vi "Main.vi"(8 "error in (no error)":errorcluster, 11 "ModuleAdmin":refnum<class "ModuleAdmin.lvclass">) -> ()   [LabVIEW 2014, in "OutputToFileModule.lvlib"]
uses:
  OutputToFileModule.lvlib
  <userlib>/NIST/ModuleAdminLib/ModuleAdmin/ModuleAdmin.lvclass
  PublicAPI/Arguments/Requests/clStopArgument.ctl
  <userlib>/NIST/ModuleAdminLib/ModuleAdmin/ModuleAdmin.lvclass/ModuleAdmin.ctl
  OutputToFilePlugins/OutputToFileBasePlugin/OutputToFileBasePlugin.lvclass
  <userlib>/NIST/BaseClasses/BasePlugin_class/BasePlugin.lvclass/BasePlugin.ctl
  OutputToFilePlugins/OutputToFileBasePlugin/OutputToFileBasePlugin.lvclass/OutputToFileBasePlugin.ctl
  EventPlugins/EventPluginBaseClass/TypeDefs/clEvtReportArray.ctl
  EventPlugins/EventPluginBaseClass/TypeDefs/clEvtReport.ctl
  NetworkImpairmentModule/PublicAPI/Arguments/Broadcasts/dblPktLoss.ctl
  NetworkImpairmentModule/PublicAPI/Arguments/Broadcasts/dblNetworkTime.ctl
  OutputToFilePlugins/OutputToFileBasePlugin/Typedefs/PmuCfgOpt.ctl
  <vilib>/Utility/error.llb/DialogType.ctl
  <userlib>/NIST/ModuleAdminLib/ModuleAdmin/Accessors/Read ShowPanel_.vi
  <userlib>/NIST/ModuleAdminLib/ModuleAdmin/Accessors/Write ShowPanel_.vi
  <userlib>/NIST/BaseClasses/BasePlugin_class/Accessors/Write PluginIniFilePath.vi
  <userlib>/NIST/BaseClasses/BasePlugin_class/Accessors/Read PluginIniFilePath.vi
  OutputToFilePlugins/OutputToFileBasePlugin/Accessors/Read clConfigOptions.vi
  OutputToFilePlugins/OutputToFileBasePlugin/Accessors/Read OutputPath.vi
  OutputToFilePlugins/OutputToFileBasePlugin/Accessors/Write clEvtReportArray.vi
  OutputToFilePlugins/OutputToFileBasePlugin/Accessors/Write PmuImpairRptArray.vi
  OutputToFilePlugins/OutputToFileBasePlugin/Accessors/Write OutputPath.vi
  OutputToFilePlugins/OutputToFileBasePlugin/Accessors/Write dblPktLoss.vi
  OutputToFilePlugins/OutputToFileBasePlugin/Accessors/Write dblNetworkTime.vi
  OutputToFilePlugins/OutputToFileBasePlugin/Accessors/Write clConfigOptions.vi
  OutputToFilePlugins/OutputToFileBasePlugin/Accessors/Read EvtRptArray.vi
  OutputToFilePlugins/OutputToFileBasePlugin/Accessors/Read PmuImpairRptArray.vi
  <userlib>/NIST/ModuleAdminLib/ModuleAdmin/Accessors/Read CloneRegRef.vi
  <vilib>/Utility/error.llb/Error Cluster From Error Code.vi
  <vilib>/Utility/file.llb/Write To Spreadsheet File (string).vi
  <vilib>/ErrorRing/Error Ring.xnode
  <userlib>/NIST/ModuleAdminLib/CloneRegistration/CloneRegistration.lvclass
  <userlib>/NIST/ModuleAdminLib/ModuleAdmin.lvlib
  <userlib>/NIST/BaseClasses/Object_class/BaseObject.lvclass
  EventPlugins/EventPluginBaseClass/EventPluginBaseClass.lvclass
  NetworkImpairmentModule/NetworkImpairmentModule.lvlib
panel:
  out "error out":errorcluster
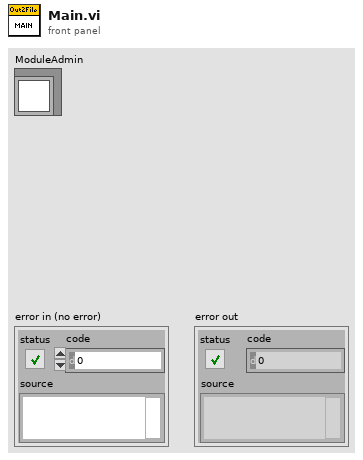
[diagram p1: front panel]
types:
  T1 = typedef "OutputToFileModule.lvlib/clRequestEvents.ctl" = cluster{"StopRequest":refnum<user-event>, "LoadPluginRequest":refnum<user-event>, "ReadPathToPluginRequest":refnum<user-event>, "WriteEvtRptRequest":refnum<user-event>, "WritePmuImpairRptRequest":refnum<user-event>, "WriteNetTimeRequest":refnum<user-event>, "WritePktLossRequest":refnum<user-event>, "WritePmuConfigRequest":refnum<user-event>, "ReadPmuConfigRequest":refnum<user-event>, "WriteOutPathRequest":refnum<user-event>, "ReadOutPathRequest":refnum<user-event>, "WriteFlagImpairRequest":refnum<user-event>, "OutputRefFileRequest":refnum<user-event>, "OutputImpairedFileRequest":refnum<user-event>, "OutputErrorDataRequest":refnum<user-event>, "OpenConfigRequest":refnum<user-event>, "ShowPanel":refnum<user-event>}
  T2 = typedef "OutputToFileModule.lvlib/clBroadcastEvents.ctl" = cluster{"DidInit":refnum<user-event>, "StatusUpdate":refnum<user-event>, "ErrorReport":refnum<user-event>, "DidStop":refnum<user-event>, "PathToPlugin":refnum<user-event>, "PmuConfig":refnum<user-event>, "OutputPath":refnum<user-event>}
  T3 = typedef "OutputToFileModule.lvlib/clStopArgument.ctl" = cluster{"Exit via Stop Module Req?":bool, "Wait for Module to stop?":bool, "ModuleAdmin":refnum<class "ModuleAdmin.lvclass">}
  T4 = enum32{"Invalid", "Standard", "Closed", "Hidden", "Minimized", "Maximized"}
  T5 = typedef "EventPlugins.lvlib/EventPluginBaseClass.lvclass/clEvtReportArray.ctl" = T6[]
  T6 = typedef "EventPlugins.lvlib/EventPluginBaseClass.lvclass/clEvtReport.ctl" = cluster{"Timestamp":dbl, "Synx":cdb[], "Freq":dbl, "ROCOF":dbl, "ID":i16}
  T7 = typedef "OutputToFilePlugins.lvlib/OutputToFileBasePlugin.lvclass/PmuCfgOpt.ctl" = cluster{"TIME_BASE":u64, "STN":string, "IDCODE":u16, "rdoPolRect":enum32{"Rectangular", "Polar"}, "rdoFloatInt":enum32{"Float", "Integer"}, "PHUNIT":u64, "rdoFreqDfreq":enum32{"Float", "Integer"}, "CHNAM":string[], "chkCfg2Prefix":bool}
  T8 = typedef "NetworkImpairmentModule.lvlib/dblPktLoss.ctl" = dbl[]
  T9 = typedef "NetworkImpairmentModule.lvlib/dblNetworkTime.ctl" = dbl[]
  T10 = typedef "DialogType.ctl" = u16
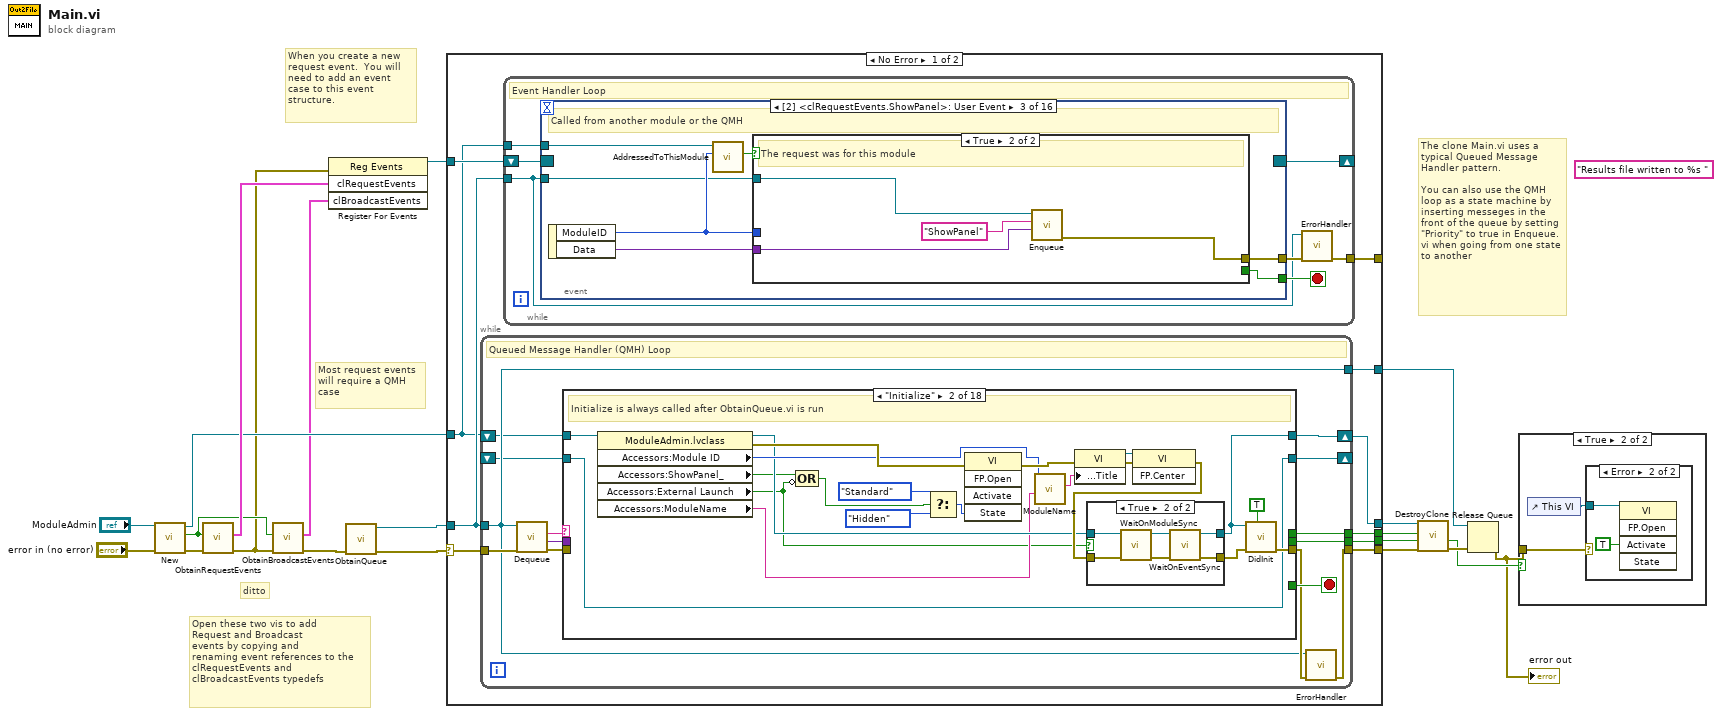
[diagram p0: block diagram]
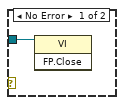
[diagram p3: hidden frame]
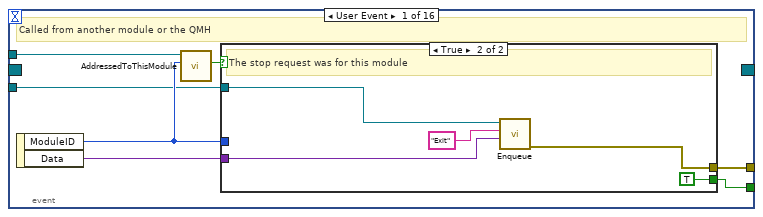
[diagram p4: hidden frame]
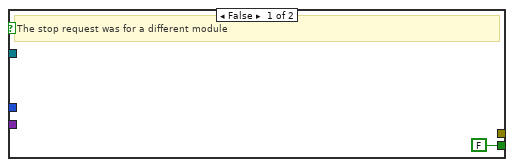
[diagram p5: hidden frame]
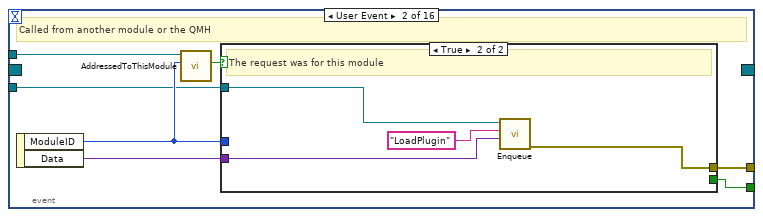
[diagram p6: hidden frame]
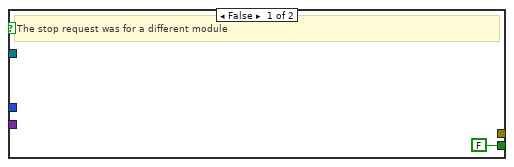
[diagram p7: hidden frame]
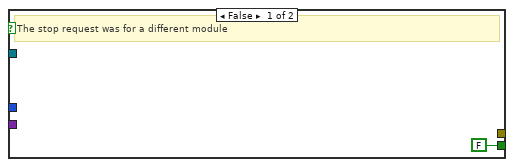
[diagram p8: hidden frame]
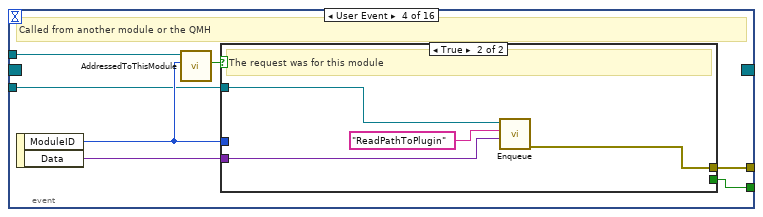
[diagram p9: hidden frame]
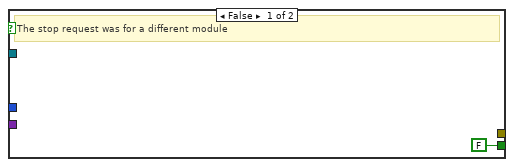
[diagram p10: hidden frame]
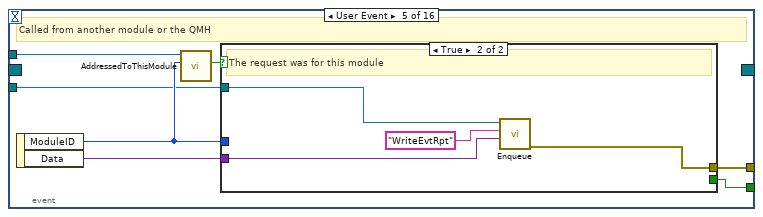
[diagram p11: hidden frame]
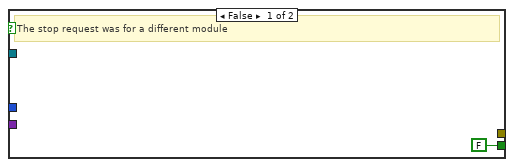
[diagram p12: hidden frame]
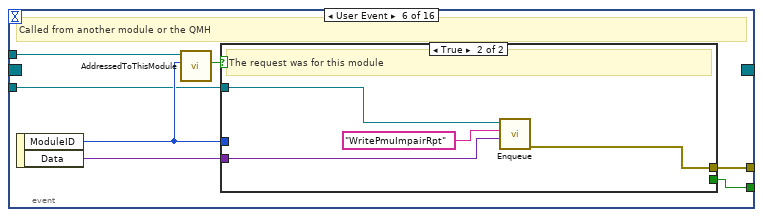
[diagram p13: hidden frame]
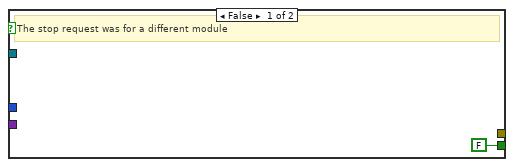
[diagram p14: hidden frame]
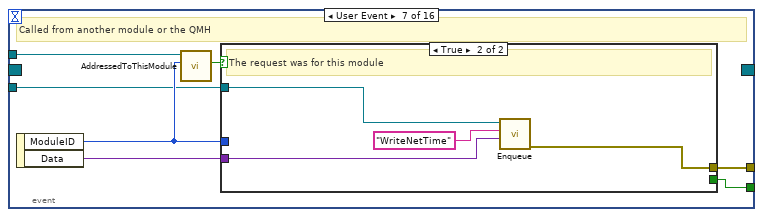
[diagram p15: hidden frame]
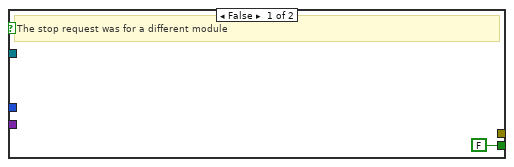
[diagram p16: hidden frame]
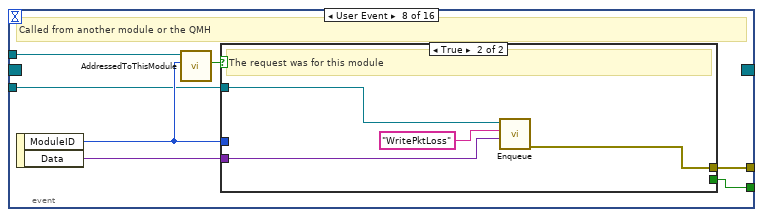
[diagram p17: hidden frame]
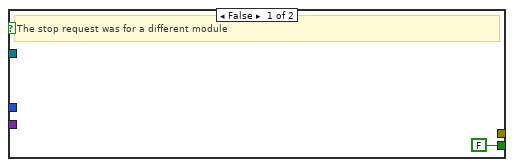
[diagram p18: hidden frame]
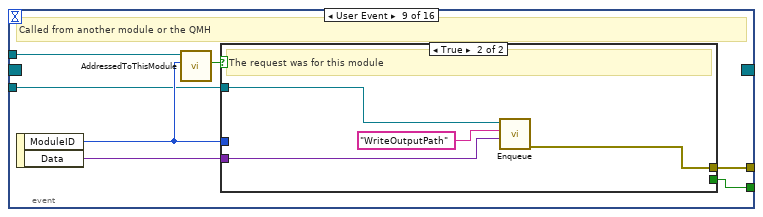
[diagram p19: hidden frame]
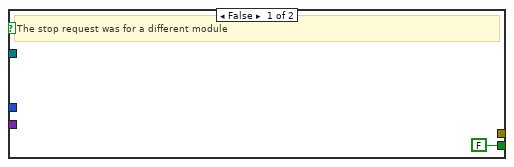
[diagram p20: hidden frame]
diagram:
  (unwired) "Results file written to %s " ("Status")
  # "The clone Main.vi uses a typical Queued Message Handler pattern.  \n\nYou can also use the QMH loop as a state machine by inserting messeges in the front of the queue by setting \"Priority\" to true in Enqueue.vi when going from one state to another"
  # "Open these two vis to add\nRequest and Broadcast \nevents by copying and \nrenaming event references to the \nclRequestEvents and \nclBroadcastEvents typedefs"
  # "ditto"
  # "Most request events\nwill require a QMH\ncase"
  # "When you create a new request event.  You will need to add an event case to this event structure."
  n1 = call <userlib>:"New.vi"("error in (no error)"="error in (no error)", "ModuleAdmin"="ModuleAdmin") -> ("error out"=w18:errorcluster, "First?"=w11:bool, "ModuleAdmin"=w14:refnum<class "ModuleAdmin.lvclass">)  [unwired: 7 in]
  n2 = call "ObtainRequestEvents.vi"("error in (no error)"=w18, "CreateNew (F)"=w11) -> ("error out"=w10:errorcluster, "clRequestEvents"=w17:T1)  [unwired: 8 in]
  n3 = call "ObtainBroadcastEvents.vi"("error in (no error)"=w10, "CreateNew? (F)"=w11) -> ("error out"=w12:errorcluster, "clBroadcastEvents"=w9:T2)  [unwired: 8 in]
  n4 = register-events(error in=w10, w17, w9) -> (reference out=w8:refnum<event-registration>)  [unwired: 1 in, 1 out]
  n5 = call "ObtainQueue.vi"("error in (no error)"=w12) -> ("error out"=w16:errorcluster, "MessageQueue"=w15:refnum<queue>)  [unwired: 9 in]
  n6 = case shown="No Error" w16 {
    selector: w16 -> [w30 w527]
    tunnel: w15 -> [w28 w523]
    tunnel: w14 -> [w25 w524]
    tunnel: [w29 w525] -> w7
    tunnel: [w27 w523] -> w13
    tunnel: w8 -> [w26 _]
    tunnel: [w24 w522] -> w5
    tunnel: [w23 _] -> w4
    tunnel: [w22 _] -> w3
    tunnel: [w21 _] -> _
    frame No Error {
      n7 = while {
        tunnel: w28 -> [w232]
        tunnel: w30 -> [w240]
        tunnel: [w234] -> w29
        tunnel: [w232] -> w27
        tunnel: [w236] -> w23
        tunnel: [w235] -> w22
        shift-right: [w231] -> _
        shift-left: _ -> [w230]
        shift-right: [w228] -> w24
        shift-left: w25 -> [w229]
        stop <- w241 stop-if-true
        # "Queued Message Handler (QMH) Loop"
        n8 = call "Dequeue.vi"("error in (no error)"=w240, "MessageQueue"=w232) -> ("error out"=w239:errorcluster, "Message Data"=w237:variant, "Message"=w238:string)  [unwired: 6 in, 1 out]
        n9 = case shown="\"Initialize\"" w238 {
          selector: w238 -> [w246 _ _ _ _ _ _ _ _ _ _ _ _ _ _ _ _ _]
          tunnel: [_ _ _ _ _ _ _ _ _ _ _ _ _ _ _ _ TRUE _] -> w241
          tunnel: w229 -> [w249 w278 w290 w302 w350 w360 w370 w383 w395 w407 w419 w431 w443 w455 w487 w489 w494 w505]
          tunnel: [w245 w267 w291 w315 w343 w354 w364 w381 w393 w405 w417 w429 w441 w453 w477 w492 w501 w506] -> w233
          tunnel: w239 -> [_ _ w293 _ w348 w358 w368 _ _ _ _ _ _ w474 w486 w493 w500 w514]
          tunnel: w237 -> [_ _ w292 w314 _ _ _ w379 w391 w403 w415 w427 w439 w475 _ _ w499 w513]
          tunnel: [_ _ _ _ _ _ _ _ _ _ _ _ _ _ _ _ w497 _] -> w236
          tunnel: [_ _ _ _ _ _ _ _ _ _ _ _ _ _ _ _ w496 _] -> w235
          tunnel: w230 -> [w243 w263 w287 w301 w351 w361 w371 w377 w390 w402 w414 w426 w438 w472 w488 w491 w495 w504]
          tunnel: [w243 w263 w287 w300 w349 w359 w369 w373 w386 w398 w411 w422 w434 w463 w484 w490 w495 w504] -> w231
          tunnel: [w242 w258 w288 w299 w342 w352 w362 w372 w384 w396 w408 w420 w432 w444 w476 w489 w494 w503] -> w228
          frame Default {
            # "Called only if a message was queued and no QMH case was created"
            n10 = property class="ModuleAdmin.lvclass"(reference=w249) -> (reference out=w242:refnum<class "ModuleAdmin.lvclass">, "Accessors:Module ID"=w248:i32, "Accessors:ModuleName"=w244:string)  [unwired: 1 in, 1 out]
            n11 = call <userlib>:"ModuleName.vi"("Name"=w244, "ModuleID"=w248) -> ("ModuleName"=w247:string)  [unwired: 9 in]
            n12 = xnode "Error Ring"("parameter 0"=w246, "parameter 1"=w247) -> ("error out"=w245:errorcluster)
          }
          frame "Initialize" {
            # "Initialize is always called after ObtainQueue.vi is run"
            n13 = property class="ModuleAdmin.lvclass"(reference=w278) -> (reference out=w264:refnum<class "ModuleAdmin.lvclass">, error out=w275:errorcluster, "Accessors:Module ID"=w266:i32, "Accessors:ShowPanel_"=w260:bool, "Accessors:External Launch"=w261:bool, "Accessors:ModuleName"=w262:string)  [unwired: 1 in]
            n14 = Compound Arithmetic op=OR(w260, invert w261) -> (w259:bool)
            n15 = Select(t=T4."Standard" ("Front Panel Window:State"), s=w259, f=T4."Hidden" ("Front Panel Window:State")) -> (s? t:f=w271:T4)
            n16 = invoke class="VI" method="FP.Open"(error in=w275, "State"=w271) -> (error out=w274:errorcluster)  [unwired: 3 in, 4 out]
            n17 = call <userlib>:"ModuleName.vi"("Name"=w262, "ModuleID"=w266) -> ("ModuleName"=w270:string)  [unwired: 9 in]
            n18 = property class="VI"(error in=w274, "Front Panel.Title"=w270) -> (reference out=w277:refnum<vi>, error out=w276:errorcluster)  [unwired: 1 in]
            n19 = invoke class="VI" method="FP.Center"(reference=w277, error in=w276) -> (error out=w265:errorcluster)  [unwired: 1 in, 2 out]
            n20 = case shown="True" w261 {
              tunnel: [w279 w285] -> w268
              tunnel: [w280 w282] -> w258
              tunnel: w265 -> [w279 w284]
              tunnel: w264 -> [w280 w281]
              frame False {
              }
              frame True {
                n21 = call <userlib>:"WaitOnModuleSync.vi"("error in (no error)"=w284, "ModuleAdmin"=w281) -> ("error out"=w286:errorcluster, "ModuleAdmin"=w283:refnum<class "ModuleAdmin.lvclass">)  [unwired: 8 in]
                n22 = call <userlib>:"WaitOnEventSync.vi"("error in (no error)"=w286, "ModuleAdmin"=w283) -> ("error out"=w285:errorcluster, "ModuleAdmin"=w282:refnum<class "ModuleAdmin.lvclass">)  [unwired: 8 in]
              }
            }
            n23 = call "DidInit.vi"("Init?"=TRUE, "error in (no error)"=w268, "ModuleAdmin"=w258) -> ("error out"=w267:errorcluster)  [unwired: 8 in]
          }
          frame "ShowPanel" {
            n24 = Variant To Data(error in=w293, type=FALSE, Variant=w292) -> (data=w289:bool, error out=w297:errorcluster)
            n25 = Select(t=T4."Standard" ("Front Panel Window:State"), s=w289, f=T4."Hidden" ("Front Panel Window:State")) -> (s? t:f=w294:T4)
            n26 = property class="VI"(error in=w297, "FP.State"=w294) -> (error out=w291:errorcluster)  [unwired: 1 in, 1 out]
            n27 = property class="ModuleAdmin.lvclass"(reference=w290, "Accessors:ShowPanel_"=w289) -> (reference out=w288:refnum<class "ModuleAdmin.lvclass">)  [unwired: 1 in, 1 out]
          }
          frame "LoadPlugin" {
            n28 = Variant To Data(type=path "", Variant=w314) -> (data=w303:path, error out=w312:errorcluster)  [unwired: 1 in]
            n29 = call <userlib>:"GetPathToClass.vi"("error in (no error)"=w312, "configuration file path"=w303) -> ("error IO"=w305:errorcluster, "PathToClass"=w311:path)  [unwired: 8 in]
            n30 = Current VI's Path() -> (path=w310:path)
            n31 = Build Path(base path=w310, name or relative path=w311) -> (appended path=w309:path)
            n32 = call <vilib>:"Check if File or Folder Exists.vi"("error in (no error)"=w305, "path"=w309) -> ("error out"=w306:errorcluster, "file or folder exists?"=w308:bool, "dup path"=w307:path)  [unwired: 7 in]
            n33 = case shown="False" w308 {
              tunnel: w307 -> [w319 w333]
              tunnel: w306 -> [w320 w330]
              tunnel: [w325 w331] -> w315
              tunnel: w301 -> [_ w329]
              tunnel: w302 -> [w322 w328]
              tunnel: [w318 w329] -> w304
              tunnel: [w316 w328] -> w299
              frame True {
                n34 = property class="ModuleAdmin.lvclass"(reference=w322) -> (reference out=w316:refnum<class "ModuleAdmin.lvclass">, "Accessors:Module ID"=w323:i32)  [unwired: 1 in, 1 out]
                n35 = call-dynamic "LoadClassFromFile.vi"("error in (no error)"=w320, "class path"=w319, "reference in"=refnum<class "OutputToFileBasePlugin.lvclass"> refnum ("OutputToFilePlugins.lvlib:OutputToFileBasePlugin.lvclass")) -> ("error out"=w324:errorcluster, "reference out"=w318:refnum<class "OutputToFileBasePlugin.lvclass">)  [unwired: 7 in]
                n36 = Path To String(path=w319) -> (string=w327:string)
                n37 = Format Into String(format string="Plugin %s  loaded", w327) -> (resulting string=w326:string)  [unwired: 2 in, 1 out]
                n38 = call "StatusUpdate.vi"("error in (no error)"=w324, "Status"=w326, "ModuleID"=w323) -> ("error out"=w325:errorcluster)  [unwired: 8 in]
              }
              frame False {
                n39 = Path To String(path=w333) -> (string=w332:string)
                n40 = xnode "Error Ring"("parameter 0"=w332) -> ("error out"=w334:errorcluster)
                n41 = Merge Errors(w334, w330) -> (w331:errorcluster)
              }
            }
            n42 = property class="OutputToFileBasePlugin.lvclass"(reference=w304, "Accessors:PluginIniFilePath"=w303) -> (reference out=w300:refnum<class "OutputToFileBasePlugin.lvclass">)  [unwired: 1 in, 1 out]
          }
          frame "ReadPathToPlugin" {
            n43 = property class="OutputToFileBasePlugin.lvclass"(reference=w351, error in=w348) -> (reference out=w349:refnum<class "OutputToFileBasePlugin.lvclass">, error out=w347:errorcluster, "Accessors:PluginIniFilePath"=w344:path)
            n44 = property class="ModuleAdmin.lvclass"(reference=w350, error in=w347) -> (reference out=w342:refnum<class "ModuleAdmin.lvclass">, error out=w346:errorcluster, "Accessors:Module ID"=w345:i32)
            n45 = call "ReadPathToPlugin.vi"("error in (no error)"=w346, "Path"=w344, "ModuleID"=w345) -> ("error out"=w343:errorcluster)  [unwired: 8 in]
          }
          frame "ReadPmuConfig" {
            n46 = property class="OutputToFileBasePlugin.lvclass"(reference=w361, error in=w358) -> (reference out=w359:refnum<class "OutputToFileBasePlugin.lvclass">, error out=w357:errorcluster, "Accessors:clConfigOptions"=w353:T7)
            n47 = property class="ModuleAdmin.lvclass"(reference=w360, error in=w357) -> (reference out=w352:refnum<class "ModuleAdmin.lvclass">, error out=w356:errorcluster, "Accessors:Module ID"=w355:i32)
            n48 = call "ReadPmuConfig.vi"("error in (no error)"=w356, "clConfigOptions"=w353, "ModuleID"=w355) -> ("error out"=w354:errorcluster)  [unwired: 8 in]
          }
          frame "ReadOutputPath" {
            n49 = property class="OutputToFileBasePlugin.lvclass"(reference=w371, error in=w368) -> (reference out=w369:refnum<class "OutputToFileBasePlugin.lvclass">, error out=w367:errorcluster, "Accessors:OutputPath"=w363:path)
            n50 = property class="ModuleAdmin.lvclass"(reference=w370, error in=w367) -> (reference out=w362:refnum<class "ModuleAdmin.lvclass">, error out=w366:errorcluster, "Accessors:Module ID"=w365:i32)
            n51 = call "ReadOutputPath.vi"("error in (no error)"=w366, "Path"=w363, "ModuleID"=w365) -> ("error out"=w364:errorcluster)  [unwired: 8 in]
          }
          frame "WriteEvtRpt" {
            n52 = Variant To Data(type=T5 [] ("clEvtReportArray"), Variant=w379) -> (data=w376:T5, error out=w375:errorcluster)  [unwired: 1 in]
            n53 = property class="OutputToFileBasePlugin.lvclass"(reference=w377, error in=w375, "Accessors:EvtRptArray"=w376) -> (reference out=w373:refnum<class "OutputToFileBasePlugin.lvclass">, error out=w374:errorcluster)
            n54 = property class="ModuleAdmin.lvclass"(reference=w383) -> (reference out=w372:refnum<class "ModuleAdmin.lvclass">, "Accessors:Module ID"=w382:i32)  [unwired: 1 in, 1 out]
            n55 = call "StatusUpdate.vi"("error in (no error)"=w374, "Status"="Event Report Received", "ModuleID"=w382) -> ("error out"=w381:errorcluster)  [unwired: 8 in]
          }
          frame "WritePmuImpairRpt" {
            n56 = Variant To Data(type=T5 [] ("clEvtReportArray"), Variant=w391) -> (data=w389:T5, error out=w388:errorcluster)  [unwired: 1 in]
            n57 = property class="OutputToFileBasePlugin.lvclass"(reference=w390, error in=w388, "Accessors:PmuImpairRptArray"=w389) -> (reference out=w386:refnum<class "OutputToFileBasePlugin.lvclass">, error out=w387:errorcluster)
            n58 = property class="ModuleAdmin.lvclass"(reference=w395) -> (reference out=w384:refnum<class "ModuleAdmin.lvclass">, "Accessors:Module ID"=w394:i32)  [unwired: 1 in, 1 out]
            n59 = call "StatusUpdate.vi"("error in (no error)"=w387, "Status"="Impair Report Received", "ModuleID"=w394) -> ("error out"=w393:errorcluster)  [unwired: 8 in]
          }
          frame "WriteOutputPath" {
            n60 = Variant To Data(type=path "", Variant=w403) -> (data=w401:path, error out=w400:errorcluster)  [unwired: 1 in]
            n61 = property class="OutputToFileBasePlugin.lvclass"(reference=w402, error in=w400, "Accessors:OutputPath"=w401) -> (reference out=w398:refnum<class "OutputToFileBasePlugin.lvclass">, error out=w399:errorcluster)
            n62 = property class="ModuleAdmin.lvclass"(reference=w407) -> (reference out=w396:refnum<class "ModuleAdmin.lvclass">, "Accessors:Module ID"=w406:i32)  [unwired: 1 in, 1 out]
            n63 = call "StatusUpdate.vi"("error in (no error)"=w399, "Status"="Output Path Received", "ModuleID"=w406) -> ("error out"=w405:errorcluster)  [unwired: 8 in]
          }
          frame "WritePktLoss" {
            w410 = T8 []  # dblPktLoss
            n64 = Variant To Data(type=w410, Variant=w415) -> (data=w409:T8, error out=w413:errorcluster)  [unwired: 1 in]
            n65 = property class="OutputToFileBasePlugin.lvclass"(reference=w414, error in=w413, "Accessors:dblPktLoss"=w409) -> (reference out=w411:refnum<class "OutputToFileBasePlugin.lvclass">, error out=w412:errorcluster)
            n66 = property class="ModuleAdmin.lvclass"(reference=w419) -> (reference out=w408:refnum<class "ModuleAdmin.lvclass">, "Accessors:Module ID"=w418:i32)  [unwired: 1 in, 1 out]
            n67 = call "StatusUpdate.vi"("error in (no error)"=w412, "Status"="Output Path Received", "ModuleID"=w418) -> ("error out"=w417:errorcluster)  [unwired: 8 in]
          }
          frame "WriteNetTime" {
            w421 = T9 []  # dblNetworkTime
            n68 = Variant To Data(type=w421, Variant=w427) -> (data=w425:T9, error out=w424:errorcluster)  [unwired: 1 in]
            n69 = property class="OutputToFileBasePlugin.lvclass"(reference=w426, error in=w424, "Accessors:dblNetworkTime"=w425) -> (reference out=w422:refnum<class "OutputToFileBasePlugin.lvclass">, error out=w423:errorcluster)
            n70 = property class="ModuleAdmin.lvclass"(reference=w431) -> (reference out=w420:refnum<class "ModuleAdmin.lvclass">, "Accessors:Module ID"=w430:i32)  [unwired: 1 in, 1 out]
            n71 = call "StatusUpdate.vi"("error in (no error)"=w423, "Status"="Net Time  Received", "ModuleID"=w430) -> ("error out"=w429:errorcluster)  [unwired: 8 in]
          }
          frame "WritePmuConfig" {
            w433 = T7 {"TIME_BASE"=1000000, "STN"="Bus_1", "IDCODE"=0, "rdoPolRect"=enum."Rectangular", "rdoFloatInt"=enum."Float", "PHUNIT"=1000000, "rdoFreqDfreq"=enum."Float", "CHNAM"=["VA", "VB", "VC", "V+", "IA", "IB", "IC", "I+"], "chkCfg2Prefix"=TRUE}  # clConfigOptions
            n72 = Variant To Data(type=w433, Variant=w439) -> (data=w437:T7, error out=w436:errorcluster)  [unwired: 1 in]
            n73 = property class="OutputToFileBasePlugin.lvclass"(reference=w438, error in=w436, "Accessors:clConfigOptions"=w437) -> (reference out=w434:refnum<class "OutputToFileBasePlugin.lvclass">, error out=w435:errorcluster)
            n74 = property class="ModuleAdmin.lvclass"(reference=w443) -> (reference out=w432:refnum<class "ModuleAdmin.lvclass">, "Accessors:Module ID"=w442:i32)  [unwired: 1 in, 1 out]
            n75 = call "StatusUpdate.vi"("error in (no error)"=w435, "Status"="Pmu Config Received", "ModuleID"=w442) -> ("error out"=w441:errorcluster)  [unwired: 8 in]
          }
          frame "OutputErrorFile" {
            n76 = Variant To Data(error in=w474, type="", Variant=w475) -> (data=w460:string, error out=w470:errorcluster)
            n77 = call "PmuErrorHdr.vi"("error in (no error)"=w470, "OutputToFile"=w472) -> ("error out"=w469:errorcluster, "ErrorHdr"=w462:string[], "OutputToFile"=w471:refnum<class "OutputToFileBasePlugin.lvclass">)  [unwired: 7 in]
            n78 = Concatenate Strings(w460, ".csv" ("string")) -> (w446:string)
            n79 = property class="OutputToFileBasePlugin.lvclass"(reference=w471, error in=w469) -> (reference out=w463:refnum<class "OutputToFileBasePlugin.lvclass">, error out=w466:errorcluster, "Accessors:EvtRptArray"=w468:T6[], "Accessors:PmuImpairRptArray"=w467:T5, "Accessors:OutputPath"=w461:path)
            n80 = call "PmuError.vi"("error in (no error)"=w466, "clPmuImpairRptArray"=w467, "clEvtReportArray"=w468) -> ("error out"=w448:errorcluster, "Results"=w465:dbl[][])  [unwired: 7 in]
            n81 = Number To Fractional String(number=w465) -> (F-format string=w464:string[][])  [unwired: 3 in]
            n82 = Build Path(base path=w461, name or relative path=w446) -> (appended path=w459:path)
            n83 = Build Array (concatenate)(w462, w464) -> (w457:string[][])
            n84 = call-poly <vilib>:"Write To Spreadsheet File.vi"("delimiter (\\t)"="," ("delimiter (\\t)"), "format (%s)"="%s" ("format (%.3f)"), "2D data"=w457, "file path (dialog if empty)"=w459) -> ("new file path (Not A Path if cancelled)"=w451:path)  [unwired: 4 in]
            n85 = property class="ModuleAdmin.lvclass"(reference=w455) -> (reference out=w444:refnum<class "ModuleAdmin.lvclass">, "Accessors:Module ID"=w454:i32)  [unwired: 1 in, 1 out]
            n86 = Path To String(path=w451) -> (string=w449:string)
            n87 = Format Into String(format string="Results file written to %s " ("Status"), error in=w448, w449) -> (resulting string=w450:string, error out=w447:errorcluster)  [unwired: 1 in]
            n88 = call "StatusUpdate.vi"("error in (no error)"=w447, "Status"=w450, "ModuleID"=w454) -> ("error out"=w453:errorcluster)  [unwired: 8 in]
          }
          frame "OutputAppInput" {
            n89 = call-dynamic "OutputAppInput.vi"("error in (no error)"=w486, "OutputToFileBasePlugin in"=w488) -> ("error out"=w480:errorcluster, "FilePath"=w485:path, "OutputToFileBasePlugin out"=w484:refnum<class "OutputToFileBasePlugin.lvclass">)  [unwired: 7 in]
            n90 = property class="ModuleAdmin.lvclass"(reference=w487) -> (reference out=w476:refnum<class "ModuleAdmin.lvclass">, "Accessors:Module ID"=w483:i32)  [unwired: 1 in, 1 out]
            n91 = Path To String(path=w485) -> (string=w479:string)
            n92 = Format Into String(format string="App Input Written To %s", error in=w480, w479) -> (resulting string=w482:string, error out=w478:errorcluster)  [unwired: 1 in]
            n93 = call "StatusUpdate.vi"("error in (no error)"=w478, "Status"=w482, "ModuleID"=w483) -> ("error out"=w477:errorcluster)  [unwired: 8 in]
          }
          frame "OpenConfig" {
            n94 = call-dynamic "OutToFileConfig.vi"("error in (no error)"=w493, "OutputToFileBasePlugin in"=w491) -> ("error out"=w492:errorcluster, "OutputToFileBasePlugin out"=w490:refnum<class "OutputToFileBasePlugin.lvclass">)  [unwired: 8 in]
          }
          frame "Exit" {
            # "Called by the StopRequest event handler case"
            n95 = control-ref of="This VI"() -> (w498:refnum<vi>)
            n96 = call "HandleExit.vi"("error in (no error)"=w500, "VI Refnum"=w498, "StopArgument"=w499, "ModuleAdmin"=w494) -> ("error out"=w501:errorcluster, "Exit via Stop Module Req?"=w496:bool, "WaitForStop?"=w497:bool)  [unwired: 5 in]
          }
          frame "Error" {
            n97 = property class="ModuleAdmin.lvclass"(reference=w505) -> (reference out=w503:refnum<class "ModuleAdmin.lvclass">, "Accessors:External Launch"=w509:bool, "Accessors:Module ID"=w507:i32)  [unwired: 1 in, 1 out]
            n98 = Variant To Data(error in=w514, type=errorcluster {"status"=FALSE, "code"=0, "source"=""} ("error constant"), Variant=w513) -> (data=w508:errorcluster, error out=w511:errorcluster)
            n99 = call "ReportError.vi"("error in (no error)"=w511, "ErrorReported"=w508, "ModuleID"=w507) -> ("error out"=w510:errorcluster)  [unwired: 8 in]
            n100 = case shown="False" w509 {
              tunnel: w510 -> [w518 w519]
              tunnel: w508 -> [w517 _]
              tunnel: [w516 w519] -> w506
              tunnel: w505 -> [w515 _]
              frame False {
                # "Todo:  Add an event to ask the user\nIf the module should stop or continue"
                # "Stand alone: now, force an exit"
                n101 = call <vilib>:"Simple Error Handler.vi"("error in (no error)"=w517) -> ()  [unwired: 4 in, 5 out]
                n102 = call "StopRequest.vi"("error in (no error)"=w518, "ModuleAdmin"=w515) -> ("error out"=w516:errorcluster)  [unwired: 8 in, 1 out]
              }
              frame True {
                # "Externally launched modules only broadcast the error msg"
              }
            }
          }
        }
        n103 = call "ErrorHandler.vi"("error in (no error)"=w233, "MessageQueue"=w232) -> ("error out"=w234:errorcluster)  [unwired: 8 in, 1 out]
      }
      n104 = while {
        tunnel: w28 -> [w31]
        shift-right: [w35] -> _
        shift-left: w26 -> [w36]
        tunnel: w25 -> [w34]
        tunnel: [w32] -> w21
        stop <- w37 stop-if-true
        # "Event Handler Loop"
        n105 = event shown="[2] <clRequestEvents.ShowPanel>: User Event" {
          selector: w36 -> [_ _ _ _ _ _ _ _ _ _ _ _ _ _ _ _]
          dyn-events: [_ _ _ _ _ _ _ _ _ _ _ _ _ _ _ _] -> w35
          timeout: _ -> [_ _ _ _ _ _ _ _ _ _ _ _ _ _ _ _]
          tunnel: w31 -> [w41 w54 w66 w78 w90 w102 w114 w126 w138 w150 w161 w171 w182 w194 w206 w227]
          tunnel: [w40 w53 w65 w77 w89 w101 w113 w125 w137 w149 w160 w170 w181 w193 w205 TRUE] -> w37
          tunnel: w34 -> [w44 w57 w69 w81 w93 w105 w117 w129 w141 w153 w164 w174 w185 w197 w209 w221]
          tunnel: [w39 w52 w64 w76 w88 w100 w112 w124 w136 w148 w159 w169 w180 w192 w204 w225] -> w33
          event User Event {
            # "Called from another module or the QMH"
            n106 = event-data() -> ("ModuleID"=w42:i32, "Data"=w38:variant)  [unwired: 1 in]
            n107 = call <userlib>:"AddressedToThisModule.vi"("ModuleID"=w42, "ModuleAdmin"=w44) -> ("AddressedToThisInstance?"=w43:bool)  [unwired: 8 in, 1 out]
            n108 = case shown="True" w43 {
              tunnel: w42 -> [_ _]
              tunnel: w41 -> [_ w50]
              tunnel: [FALSE TRUE] -> w40
              tunnel: [_ w48] -> w39
              tunnel: w38 -> [_ w46]
              frame False {
                # "The stop request was for a different module"
              }
              frame True {
                # "The stop request was for this module"
                n109 = call "Enqueue.vi"("Message Data"=w46, "Message"="Exit", "MessageQueue"=w50) -> ("error out"=w48:errorcluster)  [unwired: 7 in, 1 out]
              }
            }
          }
          event User Event {
            # "Called from another module or the QMH"
            n110 = event-data() -> ("ModuleID"=w55:i32, "Data"=w51:variant)  [unwired: 1 in]
            n111 = call <userlib>:"AddressedToThisModule.vi"("ModuleID"=w55, "ModuleAdmin"=w57) -> ("AddressedToThisInstance?"=w56:bool)  [unwired: 8 in, 1 out]
            n112 = case shown="True" w56 {
              tunnel: w55 -> [_ _]
              tunnel: w54 -> [_ w62]
              tunnel: [FALSE _] -> w53
              tunnel: [_ w61] -> w52
              tunnel: w51 -> [_ w59]
              frame False {
                # "The stop request was for a different module"
              }
              frame True {
                # "The request was for this module"
                n113 = call "Enqueue.vi"("Message Data"=w59, "Message"="LoadPlugin", "MessageQueue"=w62) -> ("error out"=w61:errorcluster)  [unwired: 7 in, 1 out]
              }
            }
          }
          event User Event {
            # "Called from another module or the QMH"
            n114 = event-data() -> ("ModuleID"=w67:i32, "Data"=w63:variant)  [unwired: 1 in]
            n115 = call <userlib>:"AddressedToThisModule.vi"("ModuleID"=w67, "ModuleAdmin"=w69) -> ("AddressedToThisInstance?"=w68:bool)  [unwired: 8 in, 1 out]
            n116 = case shown="True" w68 {
              tunnel: w67 -> [_ _]
              tunnel: w66 -> [_ w74]
              tunnel: [FALSE _] -> w65
              tunnel: [_ w73] -> w64
              tunnel: w63 -> [_ w71]
              frame False {
                # "The stop request was for a different module"
              }
              frame True {
                # "The request was for this module"
                n117 = call "Enqueue.vi"("Message Data"=w71, "Message"="ShowPanel", "MessageQueue"=w74) -> ("error out"=w73:errorcluster)  [unwired: 7 in, 1 out]
              }
            }
          }
          event User Event {
            # "Called from another module or the QMH"
            n118 = event-data() -> ("ModuleID"=w79:i32, "Data"=w75:variant)  [unwired: 1 in]
            n119 = call <userlib>:"AddressedToThisModule.vi"("ModuleID"=w79, "ModuleAdmin"=w81) -> ("AddressedToThisInstance?"=w80:bool)  [unwired: 8 in, 1 out]
            n120 = case shown="True" w80 {
              tunnel: w79 -> [_ _]
              tunnel: w78 -> [_ w86]
              tunnel: [FALSE _] -> w77
              tunnel: [_ w85] -> w76
              tunnel: w75 -> [_ w83]
              frame False {
                # "The stop request was for a different module"
              }
              frame True {
                # "The request was for this module"
                n121 = call "Enqueue.vi"("Message Data"=w83, "Message"="ReadPathToPlugin", "MessageQueue"=w86) -> ("error out"=w85:errorcluster)  [unwired: 7 in, 1 out]
              }
            }
          }
          event User Event {
            # "Called from another module or the QMH"
            n122 = event-data() -> ("ModuleID"=w91:i32, "Data"=w87:variant)  [unwired: 1 in]
            n123 = call <userlib>:"AddressedToThisModule.vi"("ModuleID"=w91, "ModuleAdmin"=w93) -> ("AddressedToThisInstance?"=w92:bool)  [unwired: 8 in, 1 out]
            n124 = case shown="True" w92 {
              tunnel: w91 -> [_ _]
              tunnel: w90 -> [_ w98]
              tunnel: [FALSE _] -> w89
              tunnel: [_ w97] -> w88
              tunnel: w87 -> [_ w95]
              frame False {
                # "The stop request was for a different module"
              }
              frame True {
                # "The request was for this module"
                n125 = call "Enqueue.vi"("Message Data"=w95, "Message"="WriteEvtRpt", "MessageQueue"=w98) -> ("error out"=w97:errorcluster)  [unwired: 7 in, 1 out]
              }
            }
          }
          event User Event {
            # "Called from another module or the QMH"
            n126 = event-data() -> ("ModuleID"=w103:i32, "Data"=w99:variant)  [unwired: 1 in]
            n127 = call <userlib>:"AddressedToThisModule.vi"("ModuleID"=w103, "ModuleAdmin"=w105) -> ("AddressedToThisInstance?"=w104:bool)  [unwired: 8 in, 1 out]
            n128 = case shown="True" w104 {
              tunnel: w103 -> [_ _]
              tunnel: w102 -> [_ w110]
              tunnel: [FALSE _] -> w101
              tunnel: [_ w109] -> w100
              tunnel: w99 -> [_ w107]
              frame False {
                # "The stop request was for a different module"
              }
              frame True {
                # "The request was for this module"
                n129 = call "Enqueue.vi"("Message Data"=w107, "Message"="WritePmuImpairRpt", "MessageQueue"=w110) -> ("error out"=w109:errorcluster)  [unwired: 7 in, 1 out]
              }
            }
          }
          event User Event {
            # "Called from another module or the QMH"
            n130 = event-data() -> ("ModuleID"=w115:i32, "Data"=w111:variant)  [unwired: 1 in]
            n131 = call <userlib>:"AddressedToThisModule.vi"("ModuleID"=w115, "ModuleAdmin"=w117) -> ("AddressedToThisInstance?"=w116:bool)  [unwired: 8 in, 1 out]
            n132 = case shown="True" w116 {
              tunnel: w115 -> [_ _]
              tunnel: w114 -> [_ w122]
              tunnel: [FALSE _] -> w113
              tunnel: [_ w121] -> w112
              tunnel: w111 -> [_ w119]
              frame False {
                # "The stop request was for a different module"
              }
              frame True {
                # "The request was for this module"
                n133 = call "Enqueue.vi"("Message Data"=w119, "Message"="WriteNetTime", "MessageQueue"=w122) -> ("error out"=w121:errorcluster)  [unwired: 7 in, 1 out]
              }
            }
          }
          event User Event {
            # "Called from another module or the QMH"
            n134 = event-data() -> ("ModuleID"=w127:i32, "Data"=w123:variant)  [unwired: 1 in]
            n135 = call <userlib>:"AddressedToThisModule.vi"("ModuleID"=w127, "ModuleAdmin"=w129) -> ("AddressedToThisInstance?"=w128:bool)  [unwired: 8 in, 1 out]
            n136 = case shown="True" w128 {
              tunnel: w127 -> [_ _]
              tunnel: w126 -> [_ w134]
              tunnel: [FALSE _] -> w125
              tunnel: [_ w133] -> w124
              tunnel: w123 -> [_ w131]
              frame False {
                # "The stop request was for a different module"
              }
              frame True {
                # "The request was for this module"
                n137 = call "Enqueue.vi"("Message Data"=w131, "Message"="WritePktLoss", "MessageQueue"=w134) -> ("error out"=w133:errorcluster)  [unwired: 7 in, 1 out]
              }
            }
          }
          event User Event {
            # "Called from another module or the QMH"
            n138 = event-data() -> ("ModuleID"=w139:i32, "Data"=w135:variant)  [unwired: 1 in]
            n139 = call <userlib>:"AddressedToThisModule.vi"("ModuleID"=w139, "ModuleAdmin"=w141) -> ("AddressedToThisInstance?"=w140:bool)  [unwired: 8 in, 1 out]
            n140 = case shown="False" w140 {
              tunnel: w139 -> [_ _]
              tunnel: w138 -> [_ w146]
              tunnel: [FALSE _] -> w137
              tunnel: [_ w145] -> w136
              tunnel: w135 -> [_ w143]
              frame False {
                # "The stop request was for a different module"
              }
              frame True {
                # "The request was for this module"
                n141 = call "Enqueue.vi"("Message Data"=w143, "Message"="WriteOutputPath", "MessageQueue"=w146) -> ("error out"=w145:errorcluster)  [unwired: 7 in, 1 out]
              }
            }
          }
          event User Event {
            # "Called from another module or the QMH"
            n142 = event-data() -> ("ModuleID"=w151:i32, "Data"=w147:variant)  [unwired: 1 in]
            n143 = call <userlib>:"AddressedToThisModule.vi"("ModuleID"=w151, "ModuleAdmin"=w153) -> ("AddressedToThisInstance?"=w152:bool)  [unwired: 8 in, 1 out]
            n144 = case shown="False" w152 {
              tunnel: w151 -> [_ _]
              tunnel: w150 -> [_ w158]
              tunnel: [FALSE _] -> w149
              tunnel: [_ w157] -> w148
              tunnel: w147 -> [_ w155]
              frame False {
                # "The stop request was for a different module"
              }
              frame True {
                # "The request was for this module"
                n145 = call "Enqueue.vi"("Message Data"=w155, "Message"="WritePmuConfig", "MessageQueue"=w158) -> ("error out"=w157:errorcluster)  [unwired: 7 in, 1 out]
              }
            }
          }
          event User Event {
            # "Called from another module or the QMH"
            n146 = event-data() -> ("ModuleID"=w162:i32)  [unwired: 1 in]
            n147 = call <userlib>:"AddressedToThisModule.vi"("ModuleID"=w162, "ModuleAdmin"=w164) -> ("AddressedToThisInstance?"=w163:bool)  [unwired: 8 in, 1 out]
            n148 = case shown="True" w163 {
              tunnel: w162 -> [_ _]
              tunnel: w161 -> [_ w168]
              tunnel: [FALSE _] -> w160
              tunnel: [_ w167] -> w159
              frame False {
                # "The request was for a different module"
              }
              frame True {
                # "The request was for this module"
                n149 = call "Enqueue.vi"("Message"="ReadPmuConfig", "MessageQueue"=w168) -> ("error out"=w167:errorcluster)  [unwired: 8 in, 1 out]
              }
            }
          }
          event User Event {
            # "Called from another module or the QMH"
            n150 = event-data() -> ("ModuleID"=w172:i32)  [unwired: 1 in]
            n151 = call <userlib>:"AddressedToThisModule.vi"("ModuleID"=w172, "ModuleAdmin"=w174) -> ("AddressedToThisInstance?"=w173:bool)  [unwired: 8 in, 1 out]
            n152 = case shown="True" w173 {
              tunnel: w172 -> [_ _]
              tunnel: w171 -> [_ w178]
              tunnel: [FALSE _] -> w170
              tunnel: [_ w177] -> w169
              frame False {
                # "The request was for a different module"
              }
              frame True {
                # "The request was for this module"
                n153 = call "Enqueue.vi"("Message"="ReadOutputPath", "MessageQueue"=w178) -> ("error out"=w177:errorcluster)  [unwired: 8 in, 1 out]
              }
            }
          }
          event User Event {
            # "Called from another module or the QMH"
            n154 = event-data() -> ("ModuleID"=w183:i32, "Data"=w179:variant)  [unwired: 1 in]
            n155 = call <userlib>:"AddressedToThisModule.vi"("ModuleID"=w183, "ModuleAdmin"=w185) -> ("AddressedToThisInstance?"=w184:bool)  [unwired: 8 in, 1 out]
            n156 = case shown="True" w184 {
              tunnel: w183 -> [_ _]
              tunnel: w182 -> [_ w190]
              tunnel: [FALSE _] -> w181
              tunnel: [_ w189] -> w180
              tunnel: w179 -> [_ w187]
              frame False {
                # "The request was for a different module"
              }
              frame True {
                # "The request was for this module"
                n157 = call "Enqueue.vi"("Message Data"=w187, "Message"="OutputErrorFile", "MessageQueue"=w190) -> ("error out"=w189:errorcluster)  [unwired: 7 in, 1 out]
              }
            }
          }
          event User Event {
            # "Called from another module or the QMH"
            n158 = event-data() -> ("ModuleID"=w195:i32, "Data"=w191:variant)  [unwired: 1 in]
            n159 = call <userlib>:"AddressedToThisModule.vi"("ModuleID"=w195, "ModuleAdmin"=w197) -> ("AddressedToThisInstance?"=w196:bool)  [unwired: 8 in, 1 out]
            n160 = case shown="True" w196 {
              tunnel: w195 -> [_ _]
              tunnel: w194 -> [_ w202]
              tunnel: [FALSE _] -> w193
              tunnel: [_ w201] -> w192
              tunnel: w191 -> [_ w199]
              frame False {
                # "The request was for a different module"
              }
              frame True {
                # "The request was for this module"
                n161 = call "Enqueue.vi"("Message Data"=w199, "Message"="OutputAppInput", "MessageQueue"=w202) -> ("error out"=w201:errorcluster)  [unwired: 7 in, 1 out]
              }
            }
          }
          event User Event {
            # "Called from another module or the QMH"
            n162 = event-data() -> ("ModuleID"=w207:i32, "Data"=w203:variant)  [unwired: 1 in]
            n163 = call <userlib>:"AddressedToThisModule.vi"("ModuleID"=w207, "ModuleAdmin"=w209) -> ("AddressedToThisInstance?"=w208:bool)  [unwired: 8 in, 1 out]
            n164 = case shown="True" w208 {
              tunnel: w207 -> [_ _]
              tunnel: w206 -> [_ w214]
              tunnel: [FALSE _] -> w205
              tunnel: [_ w213] -> w204
              tunnel: w203 -> [_ w211]
              frame False {
                # "The request was for a different module"
              }
              frame True {
                # "The request was for this module"
                n165 = call "Enqueue.vi"("Message Data"=w211, "Message"="OpenConfig", "MessageQueue"=w214) -> ("error out"=w213:errorcluster)  [unwired: 7 in, 1 out]
              }
            }
          }
          event Panel Close? {
            # "Hide on external launch"
            # "Discard the event so the QMH can complete"
            # "Called from another module or the QMH"
            n166 = event-data() -> ()  [unwired: 1 in, 1 out]
            n167 = property class="ModuleAdmin.lvclass"(reference=w221) -> ("Accessors:External Launch"=w216:bool)  [unwired: 1 in, 2 out]
            n168 = Bundle By Name(cluster=T3 {"Exit via Stop Module Req?"=FALSE, "Wait for Module to stop?"=FALSE, "ModuleAdmin"=refnum} ("Stop Argument"), "Wait for Module to stop?"=FALSE, "Exit via Stop Module Req?"=TRUE) -> (w222:T3)
            n169 = Select(t="HidePanel", s=w216, f="Exit" ("Message")) -> (s? t:f=w218:string)
            n170 = call "Enqueue.vi"("Message Data"=w222, "Message"=w218, "MessageQueue"=w227) -> ("error out"=w225:errorcluster)  [unwired: 7 in, 1 out]
            n171 = event-data("Discard?"=TRUE) -> ()  [unwired: 1 in, 1 out]
          }
        }
        n172 = call "ErrorHandler.vi"("error in (no error)"=w33, "MessageQueue"=w31) -> ("error out"=w32:errorcluster)  [unwired: 8 in, 1 out]
      }
    }
    frame Error {
      n173 = property class="ModuleAdmin.lvclass"(reference=w524) -> (reference out=w522:refnum<class "ModuleAdmin.lvclass">, "Accessors:CloneRegRef"=w521:refnum<data-value>, "Accessors:Module ID"=w520:i32)  [unwired: 1 in, 1 out]
      n174 = call <userlib>:"Remove.vi"("Module ID"=w520, "CloneRegRef"=w521) -> ("error out"=w526:errorcluster)  [unwired: 7 in, 2 out]
      n175 = flat-sequence {
        tunnel: w527 -> [w530]
        tunnel: w526 -> [_]
        tunnel: [w528] -> w525
        frame #0 {
          w529 = T10 2 items=["no dialog", "OK message", "continue or stop message", "OK message + warnings", "continue/stop + warnings"] ("type of dialog (OK msg:1)")
          n176 = call <vilib>:"Simple Error Handler.vi"("type of dialog (OK msg:1)"=w529, "error in (no error)"=w530) -> ("error out"=w528:errorcluster)  [unwired: 3 in, 4 out]
        }
      }
    }
  }
  n177 = call "DestroyClone.vi"("error in (no error)"=w7, "Exit via Stop Module Req?"=w3, "Wait for Module to stop?"=w4, "ModuleAdmin"=w5) -> ("error out"=w6:errorcluster, "External Launch"=w2:bool)  [unwired: 5 in, 1 out]
  n178 = Release Queue(queue=w13, error in (no error)=w6) -> (error out=w1:errorcluster)  [unwired: 1 in, 2 out]
  "error out" <- w1
  n179 = case shown="True" w2 {
    tunnel: w1 -> [_ w532]
    frame False {
    }
    frame True {
      n180 = control-ref of="This VI"() -> (w531:refnum<vi>)
      n181 = case shown="Error" w532 {
        tunnel: w531 -> [w533 w534]
        frame No Error {
          n182 = invoke class="VI" method="FP.Close"(reference=w533) -> ()  [unwired: 2 in, 3 out]
        }
        frame Error {
          n183 = invoke class="VI" method="FP.Open"(reference=w534, "Activate"=TRUE ("Activate?")) -> ()  [unwired: 3 in, 5 out]
        }
      }
    }
  }
